vi "Data entry form Post-Assembly.vi"(3 "Stack names":T2) -> (1 "Post-Assembly Comments Out":T1)   [LabVIEW 2021, in "Stack.lvclass"]
uses:
  Stack.lvclass
panel:
  in  "Submit":bool
  in  "Post-Assembly Comments (If Any)":T1
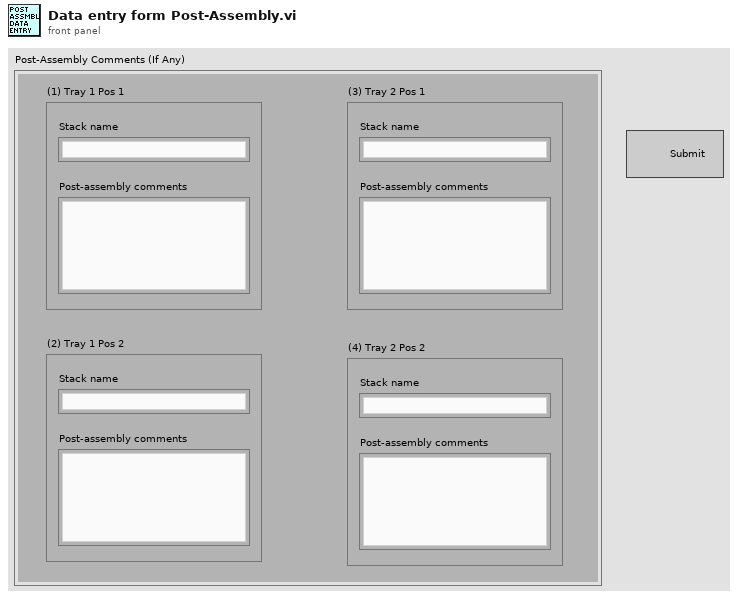
[diagram p1: front panel]
types:
  T1 = cluster{"(1) Tray 1 Pos 1":cluster{"Stack name":string, "Post-assembly comments":string}, "(2) Tray 1 Pos 2":cluster{"Stack name":string, "Post-assembly comments":string}, "(3) Tray 2 Pos 1":cluster{"Stack name":string, "Post-assembly comments":string}, "(4) Tray 2 Pos 2":cluster{"Stack name":string, "Post-assembly comments":string}}
  T2 = cluster{"(1) Tray 1 Pos 1":string, "(2) Tray 1 Pos 2":string, "(3) Tray 2 Pos 1":string, "(4) Tray 2 Pos 2":string}
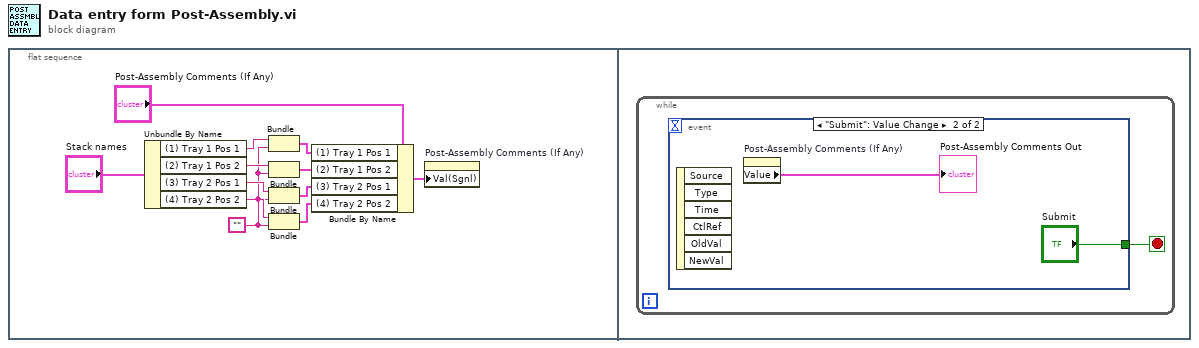
[diagram p0: block diagram]
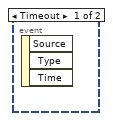
[diagram p2: hidden frame]
diagram:
  n1 = flat-sequence {
    frame #0 {
      w5 = ""
      n2 = Unbundle By Name("Stack names") -> ("(1) Tray 1 Pos 1"=w11:string, "(2) Tray 1 Pos 2"=w8:string, "(3) Tray 2 Pos 1"=w7:string, "(4) Tray 2 Pos 2"=w6:string)
      n3 = Bundle("(1) Tray 1 Pos 1"=w11, w5) -> (w10:cluster{"(1) Tray 1 Pos 1":string, string})  [unwired: 1 in]
      n4 = Bundle("(2) Tray 1 Pos 2"=w8, w5) -> (w9:cluster{"(2) Tray 1 Pos 2":string, string})  [unwired: 1 in]
      n5 = Bundle("(3) Tray 2 Pos 1"=w7, w5) -> (w4:cluster{"(3) Tray 2 Pos 1":string, string})  [unwired: 1 in]
      n6 = Bundle("(4) Tray 2 Pos 2"=w6, w5) -> (w3:cluster{"(4) Tray 2 Pos 2":string, string})  [unwired: 1 in]
      n7 = Bundle By Name(cluster="Post-Assembly Comments (If Any)", "(1) Tray 1 Pos 1"=w10, "(2) Tray 1 Pos 2"=w9, "(3) Tray 2 Pos 1"=w4, "(4) Tray 2 Pos 2"=w3) -> (w2:T1)
      n8 = property on="Post-Assembly Comments (If Any)" class="Clust (strict)"("Val(Sgnl)"=w2) -> ()  [unwired: 2 in, 2 out]
    }
    frame #1 {
      n9 = while {
        stop <- w13 stop-if-true
        n10 = event shown="[1] \"Submit\": Value Change" {
          selector: _ -> [_ _]
          dyn-events: _ -> [_ _]
          timeout: _ -> [_ _]
          tunnel: [_ "Submit"] -> w13
          event Timeout {
            n11 = event-data() -> ()  [unwired: 1 in, 3 out]
          }
          event "Submit": Value Change {
            n12 = event-data() -> ()  [unwired: 1 in, 6 out]
            n13 = property on="Post-Assembly Comments (If Any)" class="Clust (strict)"() -> ("Value"=→"Post-Assembly Comments Out":T1)  [unwired: 2 in, 2 out]
          }
        }
      }
    }
  }
